vi "DriveBegin.vi"(8 "error in (no error)":errorcluster) -> (0 "error out":errorcluster)   [LabVIEW 2025]
doc: "Begin for Drive\n\nInputs:\n -- Error in -- Error cluster -- propagated error input\n\nOutputs:\n -- Error out -- Error cluster -- progated error output"
uses:
  <vilib>/Rock Robotics/WPI/ThirdParty/JAS_Junk/TrajLib/Trajectory_Library.lvlib
  DriveGlobal.vi
  <vilib>/Rock Robotics/WPI/ThirdParty/JAS_Junk/TrajLib/TypeDef/ROTATION2D.ctl
  <vilib>/Rock Robotics/WPI/ThirdParty/JAS_Junk/TrajLib/TypeDef/SWERVE_DRIVE_MODULE_POSITION.ctl
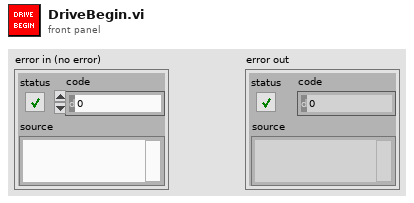
[diagram p1: front panel]
types:
  T1 = typedef "Trajectory_Library.lvlib/SWERVE_DRIVE_MODULE_POSITION.ctl" = cluster{"Distance":dbl, "Angle":T2, "P":bool}
  T2 = typedef "Trajectory_Library.lvlib/ROTATION2D.ctl" = cluster{"VALUE":dbl, "COS":dbl, "SIN":dbl}
  T3 = typedef "ADIS16470 Device Reference.ctl" = cluster{"DevStatus":errorcluster, "Hardware Config":T4, "Calibration Complete":refnum<notifier>, "Status Reference":refnum<data-value>, "Data Reference":refnum<data-value>, "Sychronous Process VI":T8, "Cmd FIFO":refnum<k33>, "Source":T9, "Data FIFO":refnum<k33>, "Calibration Time (ms)":u32, "Data Reference":refnum<data-value>}
  T4 = typedef "ADIS16470 Hardware Configuration.ctl" = cluster{"SPI Clock Rate (Hz)":dbl, "IMU SPI Mode (3)":T5, "IMU Reset Pin":T6, "IMU SPI Bus":T7, "IMU Data Ready Pin":T6, "Stall Config":cluster{"Pow2BytesPerRead":u8, "StallTicks":u16, "CsToSclkTicks":u8}}
  T5 = typedef "WPI_SPIMode.ctl" = enum16{"Mode 0 (Clk Idle Low,Sample on Leading)", "Mode 1 (Clk Idle Low,Sample on Trailing)", "Mode 2 (Clk Idle High,Sample on Leading)", "Mode 3 (Clk Idle High,Sample on Trailing)"}
  T6 = typedef "FPGA_DIOChannel.ctl" = enum8{"DIO 0", "DIO 1", "DIO 2", "DIO 3", "DIO 4", "DIO 5", "DIO 6", "DIO 7", "DIO 8", "DIO 9", "DIO MXP 0", "DIO MXP 1", "DIO MXP 2", "DIO MXP 3", "DIO MXP 4", "DIO MXP 5", "DIO MXP 6", "DIO MXP 7", "DIO MXP 8", "DIO MXP 9", "DIO MXP 10", "DIO MXP 11", "DIO MXP 12", "DIO MXP 13", "DIO MXP 14", "DIO MXP 15", "SPI Port CS1", "SPI Port CS2", "SPI Port CS3", "SPI Port MISO", "SPI Port MOSI", "Invalid"}
  T7 = typedef "spi_bus.ctl" = enum16{"SPI On-Board, CS0", "SPI On-Board, CS1", "SPI On-Board, CS2", "SPI On-Board, CS3", "SPI MXP", "Invalid"}
  T8 = typedef "ADIS16470 Process.ctl" = refnum<vi>
  T9 = typedef "FPGA_CounterEncoderSourceConvertionLVSourceType.ctl" = cluster{"DevStatus":errorcluster, "AnalogTriggerMode?":bool, "DigitalMode":cluster{"DIO Channel":T10}, "AnalogTriggerMode":cluster{"AnalogTriggerIndex":T11, "OutputType":T12}}
  T10 = typedef "FPGA_DIODigitalSourceChannel.ctl" = enum8{"DIO 0", "DIO 1", "DIO 2", "DIO 3", "DIO 4", "DIO 5", "DIO 6", "DIO 7", "DIO 8", "DIO 9", "DIO MXP 0", "DIO MXP 1", "DIO MXP 2", "DIO MXP 3", "DIO MXP 4", "DIO MXP 5", "DIO MXP 6", "DIO MXP 7", "DIO MXP 8", "DIO MXP 9", "DIO MXP 10", "DIO MXP 11", "DIO MXP 12", "DIO MXP 13", "DIO MXP 14", "DIO MXP 15", "SPI Port CS1", "SPI Port CS2", "SPI Port CS3", "SPI Port MISO", "SPI Port MOSI", "Disabled"}
  T11 = typedef "FPGA_AnalogTriggerIndex.ctl" = enum8{"Trig 0", "Trig 1", "Trig 2", "Trig 3", "Trig 4", "Trig 5", "Trig 6", "Trig 7", "Invalid"}
  T12 = typedef "FPGA_AnalogTriggerOutType.ctl" = enum16{"InWindow", "TriggerState", "Rising", "Falling"}
  T13 = typedef "Trajectory_Library.lvlib/TRANSLATION2D.ctl" = cluster{"X":dbl, "Y":dbl}
  T14 = typedef "Trajectory_Library.lvlib/SWERVE_DRIVE_KINEMATICS.ctl" = cluster{"NumModules":i32, "InverseKinematics":T15, "ForwardKinematics":T15, "Modules":T13[], "PrevCoR":T13, "SavedModuleStates":T16[]}
  T15 = typedef "NI_Matrix.lvlib/RealMatrix.ctl" = dbl[][]
  T16 = typedef "Trajectory_Library.lvlib/SWERVE_DRIVE_MODULE_STATE.ctl" = cluster{"Speed":dbl, "Angle":T2}
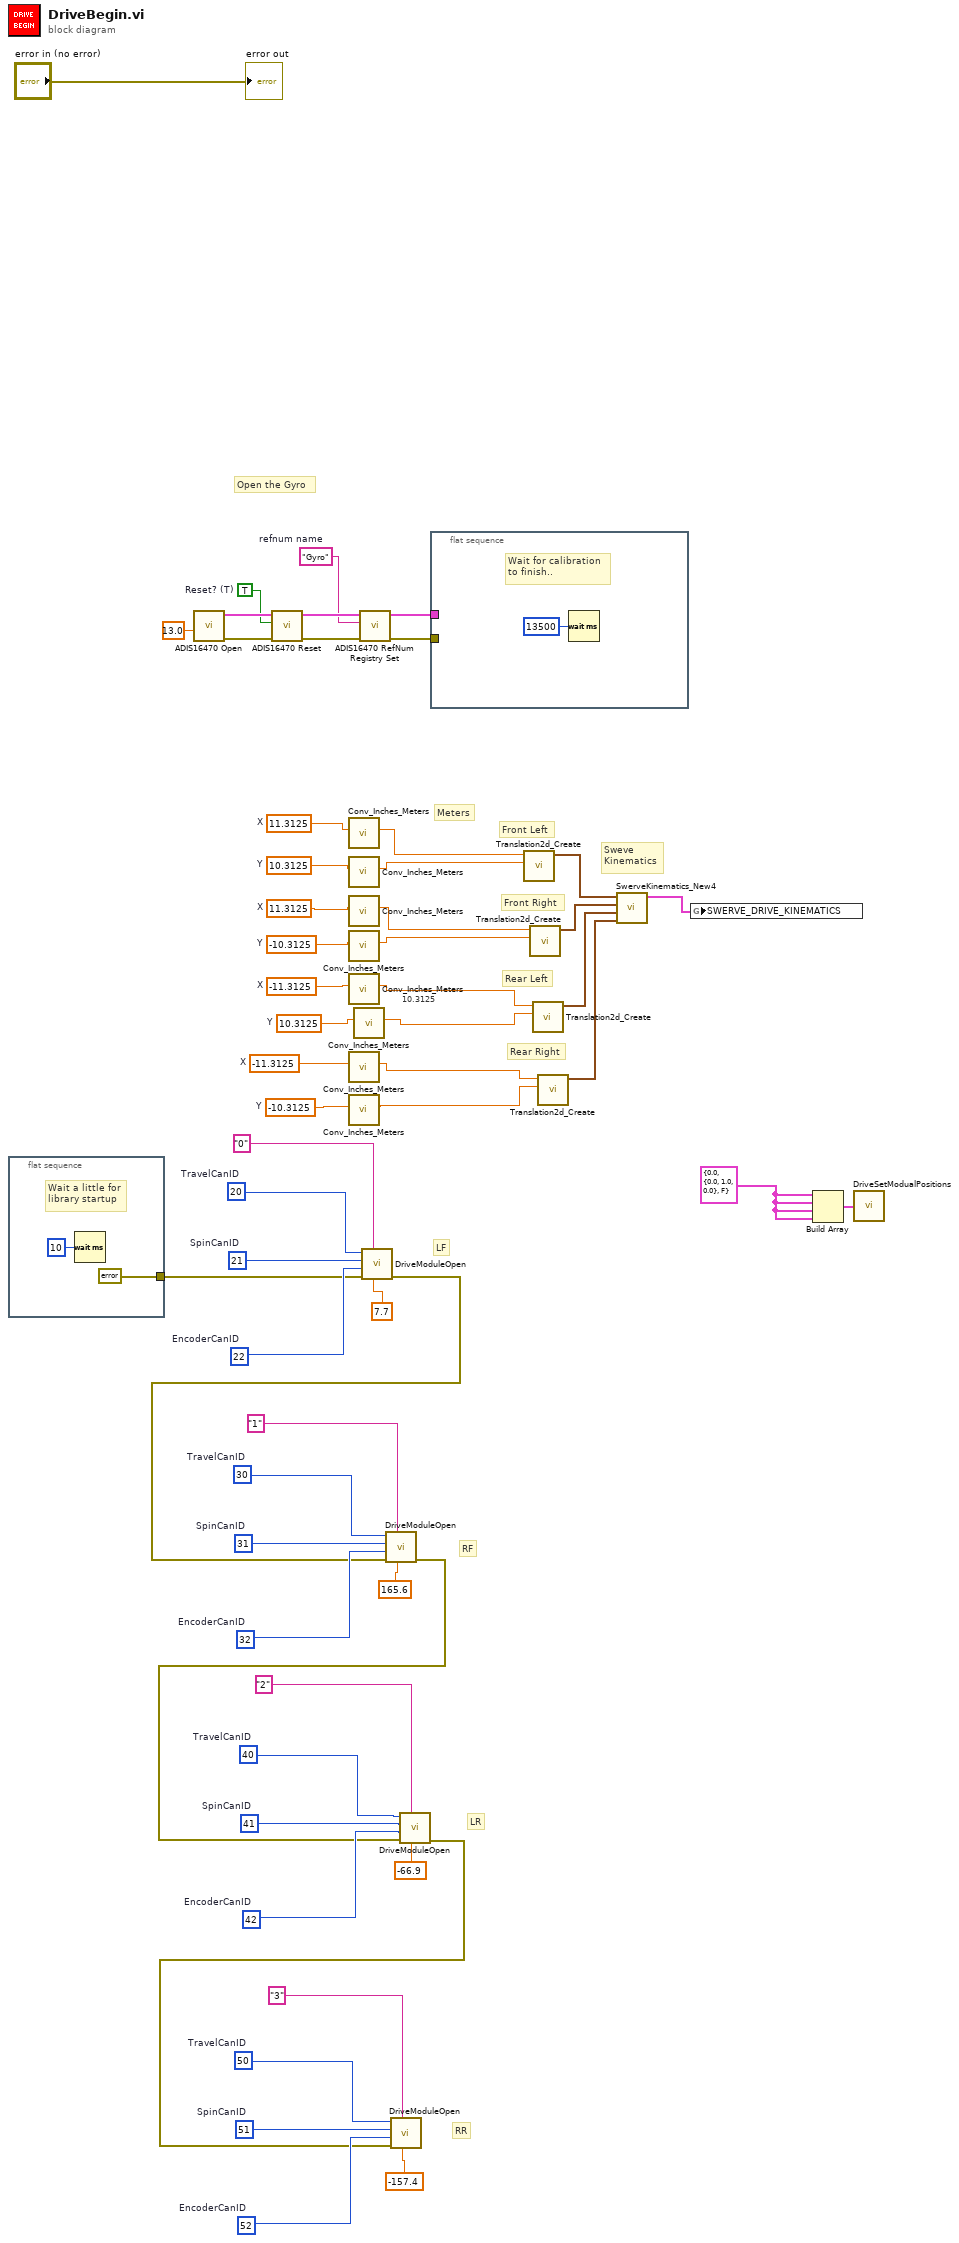
[diagram p0: block diagram]
diagram:
  w1 = T1 {"Distance"=0.0, "Angle"={"VALUE"=0.0, "COS"=1.0, "SIN"=0.0}, "P"=FALSE} ("SWERVE_DRIVE_MODULE_POSITION")
  w9 = "Gyro"  # refnum name
  w12 = TRUE  # Reset? (T)
  w22 = u8 50  # TravelCanID
  w21 = u8 51  # SpinCanID
  w20 = u8 52  # EncoderCanID
  w25 = u8 40  # TravelCanID
  w24 = u8 41  # SpinCanID
  w23 = u8 42  # EncoderCanID
  w28 = u8 30  # TravelCanID
  w27 = u8 31  # SpinCanID
  w26 = u8 32  # EncoderCanID
  w29 = u8 20  # TravelCanID
  w30 = u8 21  # SpinCanID
  w31 = u8 22  # EncoderCanID
  w38 = -11.3125  # X
  w37 = -10.3125  # Y
  w40 = -11.3125  # X
  w39 = 10.3125  # Y
  w42 = 11.3125  # X
  w41 = -10.3125  # Y
  w44 = 11.3125  # X
  w43 = 10.3125  # Y
  # "10.3125"
  # "Open the Gyro"
  # "RR"
  # "LR"
  # "RF"
  # "LF"
  # "Meters"
  # "Sweve\nKinematics"
  # "Rear Right"
  # "Rear Left"
  # "Front Right"
  # "Front Left"
  n1 = flat-sequence {
    tunnel: [errorcluster {"status"=FALSE, "code"=0, "source"=""} ("error in")] -> w3
    frame #0 {
      # "Wait a little for\nlibrary startup"
      n2 = Wait (ms)(milliseconds to wait=u32 10) -> ()  [unwired: 1 out]
    }
  }
  n3 = call <vilib>:"ADIS16470 Open.vi"("Initial Calibration Time (4s)"=13.0) -> ("error out"=w13:errorcluster, "ADIS16470DevRef"=w14:T3)  [unwired: 9 in]
  n4 = call <vilib>:"ADIS16470 Reset.vi"("error in (no error)"=w13, "Reset? (T)"=w12, "ADIS16470DevRef"=w14) -> ("error out"=w10:errorcluster, "ADIS16470DevRef"=w11:T3)  [unwired: 7 in]
  n5 = call <vilib>:"Conv_Inches_Meters.vi"("INCH"=w44) -> ("Meters"=w45:dbl)  [unwired: 10 in]
  n6 = call <vilib>:"Conv_Inches_Meters.vi"("INCH"=w43) -> ("Meters"=w46:dbl)  [unwired: 10 in]
  n7 = call <vilib>:"Conv_Inches_Meters.vi"("INCH"=w42) -> ("Meters"=w47:dbl)  [unwired: 10 in]
  n8 = call <vilib>:"Conv_Inches_Meters.vi"("INCH"=w41) -> ("Meters"=w48:dbl)  [unwired: 10 in]
  n9 = call <vilib>:"Conv_Inches_Meters.vi"("INCH"=w40) -> ("Meters"=w49:dbl)  [unwired: 10 in]
  n10 = call <vilib>:"Conv_Inches_Meters.vi"("INCH"=w38) -> ("Meters"=w52:dbl)  [unwired: 10 in]
  n11 = call <vilib>:"Conv_Inches_Meters.vi"("INCH"=w37) -> ("Meters"=w51:dbl)  [unwired: 10 in]
  n12 = call <vilib>:"Conv_Inches_Meters.vi"("INCH"=w39) -> ("Meters"=w50:dbl)  [unwired: 10 in]
  n13 = call <vilib>:"ADIS16470 RefNum Registry Set.vi"("error in (no error)"=w10, "refnum name"=w9, "ADIS16470DevRef in"=w11) -> ("error out"=w7:errorcluster, "ADIS16470DevRef out"=w8:T3)  [unwired: 7 in]
  n14 = call "DriveModuleOpen.vi"("Magnet Offset (Degrees)"=7.7, "ModualNamePrefix"="0", "error in"=w3, "EncoderCanID"=w31, "SpinCanID"=w30, "TravelCanID"=w29) -> ("error out"=w6:errorcluster)  [unwired: 5 in]
  n15 = call "DriveModuleOpen.vi"("Magnet Offset (Degrees)"=165.6, "ModualNamePrefix"="1", "error in"=w6, "EncoderCanID"=w26, "SpinCanID"=w27, "TravelCanID"=w28) -> ("error out"=w5:errorcluster)  [unwired: 5 in]
  n16 = call "DriveModuleOpen.vi"("Magnet Offset (Degrees)"=-66.9, "ModualNamePrefix"="2", "error in"=w5, "EncoderCanID"=w23, "SpinCanID"=w24, "TravelCanID"=w25) -> ("error out"=w4:errorcluster)  [unwired: 5 in]
  n17 = call "DriveModuleOpen.vi"("Magnet Offset (Degrees)"=-157.4, "ModualNamePrefix"="3", "error in"=w4, "EncoderCanID"=w20, "SpinCanID"=w21, "TravelCanID"=w22) -> ()  [unwired: 5 in, 1 out]
  n18 = flat-sequence {
    tunnel: w8 -> [_]
    tunnel: w7 -> [_]
    frame #0 {
      # "Wait for calibration\nto finish.."
      n19 = Wait (ms)(milliseconds to wait=u32 13500) -> ()  [unwired: 1 out]
    }
  }
  n20 = call <vilib>:"Translation2d_Create.vi"("Y"=w46, "X"=w45) -> ("TRANSLATION"=w53:T13)  [unwired: 9 in]
  n21 = call <vilib>:"Translation2d_Create.vi"("Y"=w48, "X"=w47) -> ("TRANSLATION"=w54:T13)  [unwired: 9 in]
  n22 = call <vilib>:"Translation2d_Create.vi"("Y"=w50, "X"=w49) -> ("TRANSLATION"=w55:T13)  [unwired: 9 in]
  n23 = call <vilib>:"Translation2d_Create.vi"("Y"=w51, "X"=w52) -> ("TRANSLATION"=w56:T13)  [unwired: 9 in]
  n24 = call <vilib>:"SwerveKinematics_New4.vi"("wheel 3"=w56, "wheel 2"=w55, "wheel 1"=w54, "wheel 0"=w53) -> ("SWERVE_DRIVE_KINEMATICS"=w36:T14)  [unwired: 7 in]
  n25 = global write "DriveGlobal.vi" "SWERVE_DRIVE_KINEMATICS"(w36) -> ()
  n26 = Build Array(w1, w1, w1, w1) -> (w2:T1[])
  n27 = call "DriveSetModualPositions.vi"("Swerve_Drive_Modual_Position"=w2) -> ()  [unwired: 11 in]
  "error out" <- "error in (no error)"
